vi "AnalySelectDecayPhosphoAndSystem.vi"(1 "Raw Data Image":T1, 5 "Pulses matrice":i32[](array[numeric]), 9 "Skip samples":i32=12, 11 "Last samples":i32=5, 12 "Scan rate (Hz)":dbl, 14 "N samples/decay":i32=150) -> (2 "Standard error Tau (us)":dbl=8.774972224805227 format="%#_3g", 3 "mean and fit":dbl[][](graph), 4 "Tau (us)":dbl=8.774972224805227 format="%#_3g", 6 "amplitude":dbl=1.3790672561842066 caption="Amplitude (au)" format="%#_3g", 10 "Residu (au)":dbl=8.774972224805227 format="%#_3g", 13 "Standard error Amplitude":dbl=8.774972224805227 format="%#_3g", 15 "Area (au)":dbl=8.774972224805227 format="%#_3g")   [LabVIEW 2013]
uses:
  <vilib>/vision/Image Controls.llb/IMAQ Image.ctl
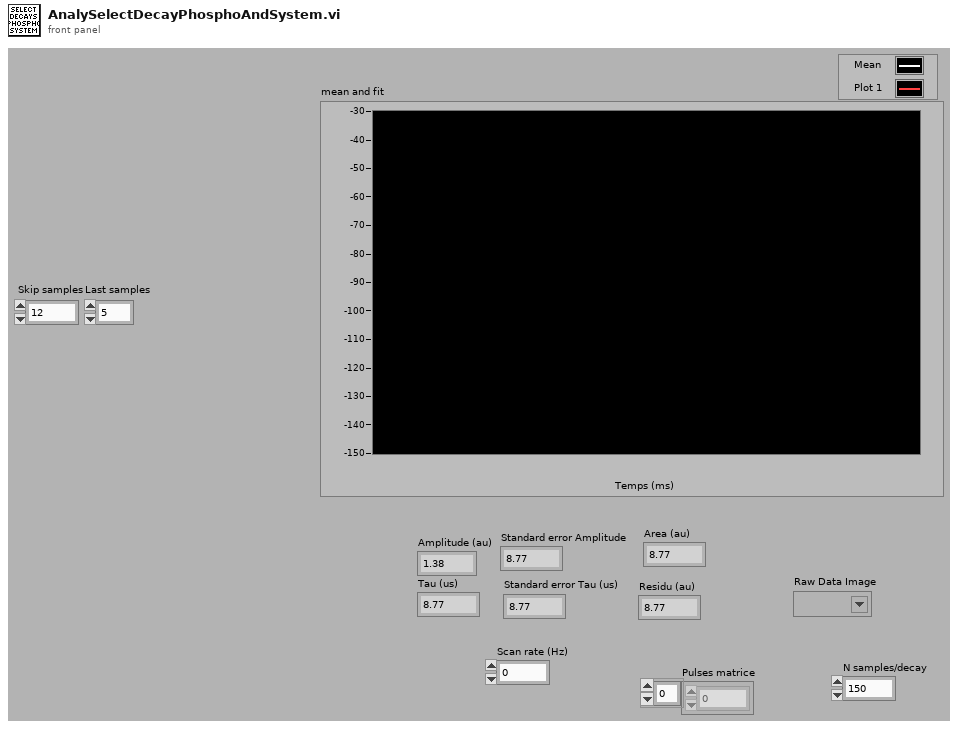
[diagram p1: front panel]
types:
  T1 = typedef "IMAQ Image.ctl" = refnum<image>
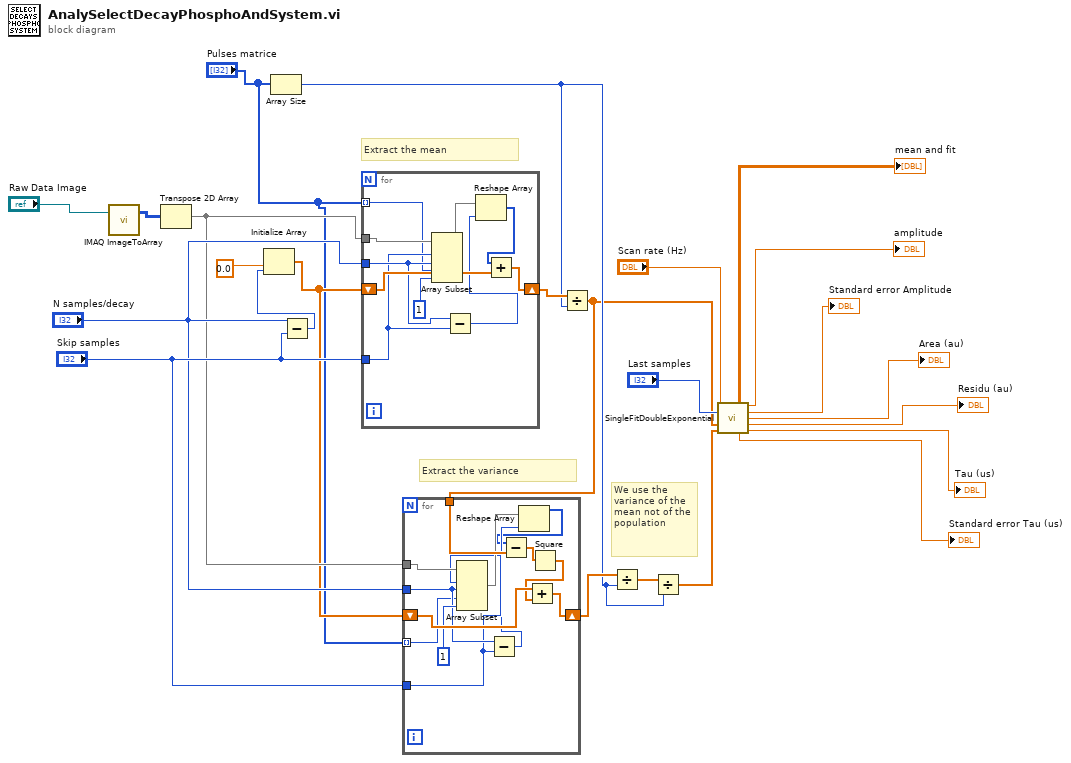
[diagram p0: block diagram]
diagram:
  # "We use the variance of the mean not of the population"
  # "Extract the variance"
  # "Extract the mean"
  n1 = call "IMAQ ImageToArray"("Image"="Raw Data Image") -> ("Image Pixels (I16)"=w17:i16[][])  [unwired: 2 in, 5 out]
  n2 = Transpose 2D Array(2D array=w17) -> (transposed array=w16:i16[][])
  n3 = Array Size(array="Pulses matrice") -> (size(s)=w3:i32)
  n4 = Subtract(x="N samples/decay", y="Skip samples") -> (x-y=w14:i32)
  n5 = Initialize Array(0.0 ("élément"), w14) -> (w15:dbl[])
  n6 = for {
    tunnel: w16 -> [w34]
    tunnel: "Skip samples" -> [w27]
    shift-right: [w31] -> w23
    shift-left: w15 -> [w32]
    tunnel: "N samples/decay" -> [w28]
    tunnel: "Pulses matrice" -> [w25] mode=indexing
    n7 = Array Subset(array=w34, index (row)=w27, length (row)=w28, index (col)=w25, length (col)=1 ("longueur")) -> (w33:i16[][])
    n8 = Subtract(x=w28, y=w27) -> (x-y=w26:i32)
    n9 = Reshape Array(w33, w26) -> (w29:i16[])
    n10 = Add(x=w29, y=w32) -> (x+y=w31:dbl[])
  }
  n11 = Divide(x=w23, y=w3) -> (x/y=w1:dbl[])
  n12 = for {
    tunnel: w16 -> [w47]
    tunnel: "Skip samples" -> [w38]
    shift-right: [w45] -> w21
    shift-left: w15 -> [w46]
    tunnel: "N samples/decay" -> [w39]
    tunnel: w1 -> [w44]
    tunnel: "Pulses matrice" -> [w35] mode=indexing
    n13 = Array Subset(array=w47, index (row)=w38, length (row)=w39, index (col)=w35, length (col)=1 ("longueur")) -> (w40:i16[][])
    n14 = Subtract(x=w39, y=w38) -> (x-y=w37:i32)
    n15 = Reshape Array(w40, w37) -> (w36:i16[])
    n16 = Subtract(x=w36, y=w44) -> (x-y=w43:dbl[])
    n17 = Square(x=w43) -> (x^2=w42:dbl[])
    n18 = Add(x=w46, y=w42) -> (x+y=w45:dbl[])
  }
  n19 = Divide(x=w21, y=w3) -> (x/y=w20:dbl[])
  n20 = Divide(x=w20, y=w3) -> (x/y=w13:dbl[])
  n21 = call "SingleFitDoubleExponential.vi"("Scan rate (Hz)"="Scan rate (Hz)", "Last point to average for baseline"="Last samples", "Input decay"=w1, "Input Variance"=w13) -> ("mean and fit"=→"mean and fit":dbl[][], "amplitude"=→"amplitude":dbl, "Standard error Amplitude"=→"Standard error Amplitude":dbl, "Area (au)"=→"Area (au)":dbl, "Residu (au)"=→"Residu (au)":dbl, "Standard error Tau (us)"=→"Standard error Tau (us)":dbl, "Tau (us)"=→"Tau (us)":dbl)  [unwired: 5 in]
